vi "Delete temp config.vi"(8 "error in (no error)":errorcluster, 11 "Config in":path) -> (0 "error out":errorcluster)   [LabVIEW 2011]
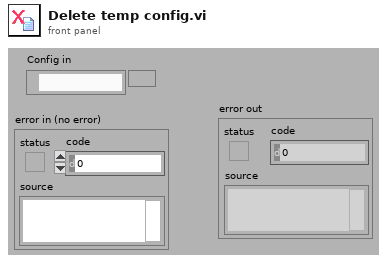
[diagram p1: front panel]
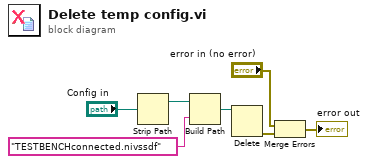
[diagram p0: block diagram]
diagram:
  n1 = Strip Path(path="Config in") -> (stripped path=w6:path)  [unwired: 1 out]
  n2 = Build Path(base path=w6, name or relative path="TESTBENCHconnected.nivssdf") -> (appended path=w4:path)
  n3 = Delete(path (use dialog)=w4) -> (error out=w2:errorcluster)  [unwired: 4 in, 2 out]
  n4 = Merge Errors("error in (no error)", w2) -> (→"error out":errorcluster)
